vi "Write Image path.vi"(8 "error in (no error)":errorcluster, 10 "Image path":path, 11 "MessageBox.lvclass in":refnum<class "MessageBox.lvclass">) -> (0 "error out":errorcluster, 3 "MessageBox.lvclass out":refnum<class "MessageBox.lvclass">)   [LabVIEW 2012, in "MessageBox.lvlib" / "MessageBox.lvclass"]
uses:
  MessageBox.lvclass
  MessageBox.lvclass/MessageBox.ctl
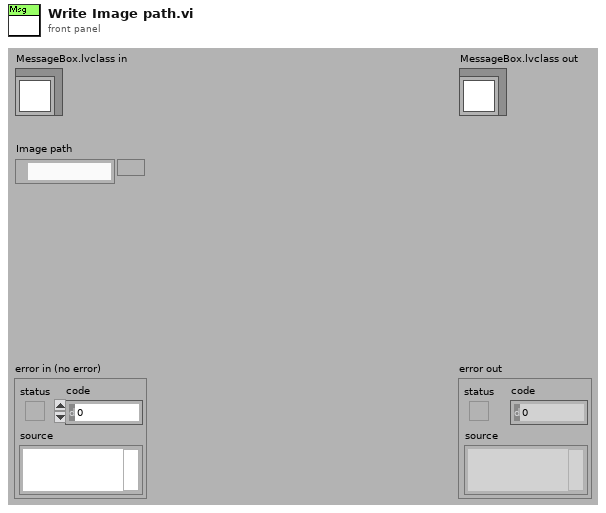
[diagram p1: front panel]
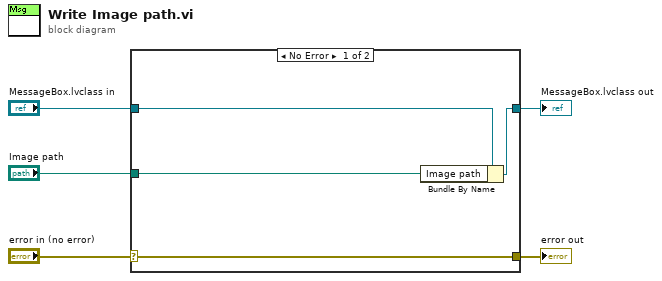
[diagram p0: block diagram]
diagram:
  n1 = case shown="No Error" "error in (no error)" {
    selector: "error in (no error)" -> [w9 w10]
    tunnel: [w9 w10] -> w4
    tunnel: [w7 w11] -> w2
    tunnel: "MessageBox.lvclass in" -> [w8 w11]
    tunnel: "Image path" -> [w6 _]
    frame No Error {
      n2 = Bundle By Name(cluster=w8, "Image path"=w6) -> (w7:refnum<class "MessageBox.lvclass">)
    }
    frame Error {
    }
  }
  "error out" <- w4
  "MessageBox.lvclass out" <- w2
